vi "Requests.vi"(8 "error in (no error)":errorcluster, 9 "write enable":bool=TRUE, 11 "ICPCON ET-7018 in":refnum<class "ICPCON ET-7018i.lvclass">) -> (0 "error out":errorcluster, 3 "ICPCON ET-7018 out":refnum<class "ICPCON ET-7018i.lvclass">)   [LabVIEW 2021, in "ICPCON ET-7018i.lvclass"]
uses:
  ICPCON ET-7018i.lvclass
  D:/my_projects/projects/Algorithms/Labview/21/Modbus/MB_TCP2/MB_TCP.lvclass
  MB_TCP.lvclass/MB_TCP.ctl
  NI_modbus_upd/Ctl/Unit_ID.ctl
  NI_modbus_upd/TCP/TCP.lvclass/TCP.ctl
  NI_modbus_upd/Master Function Definition/Responses/Read Input Registers Response.vi
  NI_modbus_upd/Master network read write.vi
  NI_modbus_upd/Master Function Definition/Requests/Read Input Registers Request.vi
  NI_modbus_upd/Master Function Definition/Responses/Read Coils Response.vi
  NI_modbus_upd/Master Function Definition/Requests/Read Coils Request.vi
  NI_modbus_upd/Utility/Bytes to U16s1.vi
  NI_modbus_upd/Function code mismatch error1.vi
  NI_modbus_upd/Error Generator1.vi
  NI_modbus_upd/Read ADU Packet Master.vi
  NI_modbus_upd/Write ADU Packet Master.vi
  NI_modbus_upd/Modbus Data Unit (PDU)/Construct PDU1.vi
  NI_modbus_upd/Utility/Bytes to Bits1.vi
  NI_modbus_upd/Modbus Data Unit (PDU)/Unflatten to PDU1.vi
  NI_modbus_upd/TCP/Protocol Read.vi
  NI_modbus_upd/TCP/Protocol Write.vi
  <vilib>/Utility/error.llb/Clear Errors.vi
  NI_modbus_upd/Modbus Data Unit (PDU)/Deconstruct PDU1.vi
  NI_modbus_upd/TCP/TCP.lvclass
  ICPCON Registers/ICPCON Registers.lvlib
  MB_TCP.lvclass
  NI_modbus_upd/NI_modbus_upd.lvlib
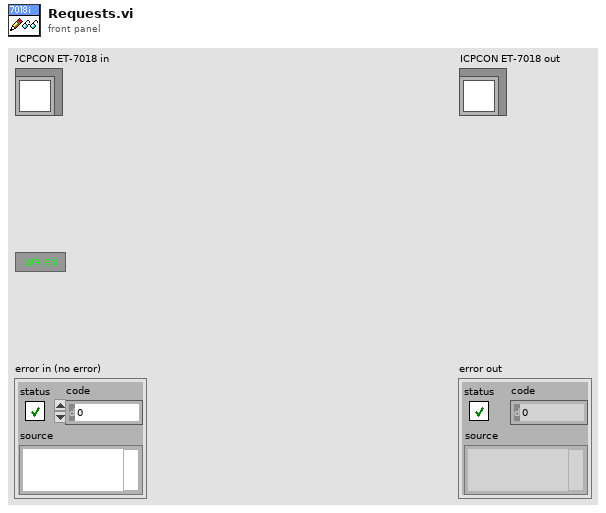
[diagram p1: front panel]
types:
  T1 = typedef "NI_modbus_upd.lvlib/Unit_ID.ctl" = cluster{"Protocol ID":u16, "Unit ID":u8}
  T2 = typedef "ICPCON Registers.lvlib/ICPCON Data.ctl" = cluster{"UTF":refnum<data-value>, "DI":refnum<data-value>, "DW":refnum<data-value>, "DO":refnum<data-value>, "IR":refnum<data-value>, "WR":refnum<data-value>, "OR":refnum<data-value>, "modified":refnum<data-value>}
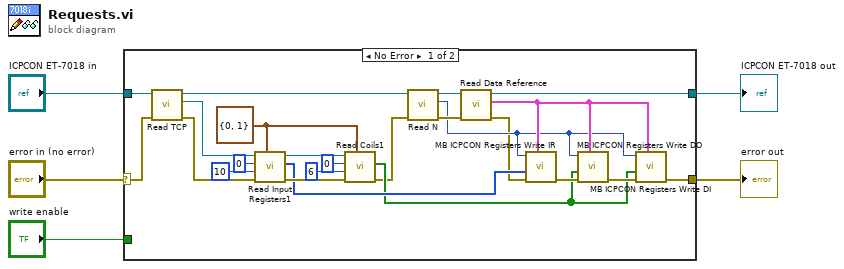
[diagram p0: block diagram]
diagram:
  n1 = case shown="No Error" "error in (no error)" {
    selector: "error in (no error)" -> [w22 w31]
    tunnel: [w24 w31] -> w3
    tunnel: [w20 w30] -> w4
    tunnel: "ICPCON ET-7018 in" -> [w23 w30]
    tunnel: "write enable" -> [_ _]
    frame No Error {
      w14 = T1 {"Protocol ID"=0, "Unit ID"=1} ("Unit_ID")
      n2 = call "Read TCP.vi"("error in (no error)"=w22, "MB_TCP in"=w23) -> ("error out"=w16:errorcluster, "TCP"=w19:refnum<class "TCP.lvclass">, "MB_TCP out"=w21:refnum<class "ICPCON ET-7018i.lvclass">)  [unwired: 7 in]
      n3 = call "Read Input Registers1.vi"("Unit_ID"=w14, "error in (no error)"=w16, "number of input registers"=u16 10, "starting address"=u16 0, "Modbus master in"=w19) -> ("error out"=w13:errorcluster, "register values"=w12:u16[], "Modbus master out"=w15:refnum<class "TCP.lvclass">)  [unwired: 4 in]
      n4 = call "Read Coils1.vi"("Unit_ID"=w14, "error in (no error)"=w13, "number of coils"=u16 6 ("number of input registers"), "starting address"=u16 0, "Modbus master in"=w15) -> ("error out"=w9:errorcluster, "coil values"=w10:bool[])  [unwired: 4 in, 1 out]
      n5 = call "Read N.vi"("error in (no error)"=w9, "MB_TCP in"=w21) -> ("error out"=w29:errorcluster, "N"=w11:i32, "MB_TCP out"=w28:refnum<class "ICPCON ET-7018i.lvclass">)  [unwired: 7 in]
      n6 = call "Read Data Reference.vi"("error in (no error)"=w29, "MB_TCP in"=w28) -> ("error out"=w8:errorcluster, "Data"=w25:T2, "MB_TCP out"=w20:refnum<class "ICPCON ET-7018i.lvclass">)  [unwired: 7 in]
      n7 = call "MB ICPCON Registers Write IR.vi"("Data Reference"=w25, "error in (no error)"=w8, "Words In"=w12, "N"=w11) -> ("error out"=w27:errorcluster)  [unwired: 7 in]
      n8 = call "MB ICPCON Registers Write DO.vi"("Data Reference"=w25, "error in (no error)"=w27, "Bits In"=w10, "N"=w11) -> ("error out"=w26:errorcluster)  [unwired: 7 in]
      n9 = call "MB ICPCON Registers Write DI.vi"("Data Reference"=w25, "error in (no error)"=w26, "Bits In"=w10, "N"=w11) -> ("error out"=w24:errorcluster)  [unwired: 7 in]
    }
    frame Error {
    }
  }
  "error out" <- w3
  "ICPCON ET-7018 out" <- w4
